vi "FT-IR Kalibrieren Linearisierung.vi"(6 "Kalibrier Optionen:":enum32{"Gasteiler", "ohne Gasteiler", "PNS"}(ring), 9 "Sprachliste":string[][](array[string]), 10 "reference (Eingang)":refnum<vi>, 11 "String (Eingang)":refnum<vi>) -> ()   [LabVIEW 2020, in "Linearisierung v2.lvlib"]
uses:
  Linearisierung v2.lvlib
  Gasteiler/Aktionen FGV Gasteiler Daten.ctl
  Gasteiler/AK-Komm Gasteiler/Aktionen AK Komm.ctl
  Aktion Lin Daten aufarbeiten.ctl
  Gasteiler/Horiba/Aktion Befehl.ctl
  Gasteiler/AK-Komm Gasteiler/Alter Gasteiler/Aktionen AK Komm_ALT.ctl
  Funktionstasten/Funktionstasten-Aktion.ctl
  Funktionstasten/Zustaende.ctl
  Sprachverwaltung/Sprachverwaltung.lvlib
  Gasteiler/Gasteiler.lvlib
  Gasteiler/AK-Komm Gasteiler/AK Komm Gasteiler.lvlib
  Gasteiler/Horiba/Horiba GDC.lvlib
  Gasteiler/AK-Komm Gasteiler/Alter Gasteiler/Alter Gasteiler.lvlib
  Funktionstasten/Funktionstasten.lvlib
  Allgemein/allgemeine Sub-VIs.lvlib
  Gasteiler/HovaCAL_Interface/Kommunikation/Kommunikation.lvlib
  Gasteiler/HovaCAL_Interface/Helper/Helper.lvlib
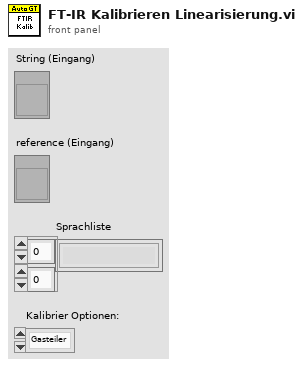
[diagram p1: front panel]
types:
  T1 = typedef "Linearisierung v2.lvlib/Gasteiler.lvlib/Aktionen FGV Gasteiler Daten.ctl" = enum16{"lesen", "Gasteiler Daten", "Seriellen Param.", "MB-Endwert", "laden", "speichern", "Anforderung", "TCP", "Aufzeichnung Start"}
  T2 = typedef "Linearisierung v2.lvlib/Gasteiler.lvlib/AK Komm Gasteiler.lvlib/Aktionen AK Komm.ctl" = enum16{"lesen", "initialisieren", "beenden", "Status", "SMAN", "SREM", "STBY", "ASTF", "ASTZ", "SLST", "AGAT", "EGAK", "AGAK", "AKAK", "ADRU", "SKOP", "SVSA", "SVSZ", "SONO", "SAIR", "SNOX", "ANOX", "SSPL", "SRUC", "SLIN", "ALST", "ETYP", "SVIO", "LCYL", "CCYL", "DCYL", "SCYL", "GCYL", "DRGV", "DRDC"}
  T3 = typedef "Linearisierung v2.lvlib/Aktion Lin Daten aufarbeiten.ctl" = enum16{"lesen", "Protkolldaten", "speichern", "laden", "EPA auswerten", "Tabelle schreiben", "Lin auswerten", "Tab init", "Stufentabelle", "EPA aktiviert", "Nachbehandlung laden", "Tabelle löschen", "Istwerte löschen", "Zeile löschen", "Zeile einfügen", "LIN aktiviert", "LIN/EPA aktiv laden", "EGAK Tab", "LIN übernehmen", "Tab init ohne Stufen"}
  T4 = typedef "Linearisierung v2.lvlib/Gasteiler.lvlib/Horiba GDC.lvlib/Aktion Befehl.ctl" = enum16{"lesen", "initialisieren", "Beenden", "Standby", "GD/CC", "Info", "Flow", "Alarm", "GD parameter", "GD point", "Durchfluss", "Spuelen1", "Spuelen1 On", "Spuelen1Off", "Spuelen2", "Ventil-Abfrage", "Reset"}
  T5 = typedef "Linearisierung v2.lvlib/Gasteiler.lvlib/AK Komm Gasteiler.lvlib/Alter Gasteiler.lvlib/Aktionen AK Komm_ALT.ctl" = enum16{"lesen", "initialisieren", "beenden", "SRES", "STBY", "SREM", "SMAN", "SLIN", "SLCH", "SLST", "SSPL", "AGAT", "ALST", "ASTZ", "ASTF", "AGAK", "EGAK"}
  T6 = typedef "Funktionstasten.lvlib/Funktionstasten-Aktion.ctl" = enum16{"Initialisieren", "Zustand setzen", "Taste gedrückt", "Fehler speichern", "Lesen", "Manuell", "Remote", "Bitparallel", "Samplepoint", "Zeit Prüfen", "reset Umschalten"}
  T7 = typedef "Funktionstasten.lvlib/Zustaende.ctl" = enum16{"Standby", "Pause", "Eco", "Messen", "Kalibrieren", "Spülen Filter", "Spülen Leitung", "Umgebungsluft", "0-Gas", "Cal-Gas", "CG zu PNS", "-------------", "Init 1", "Init 2", "Init 3", "Init 4", "Messen vorbereiten", "Messen durchführen", "Exit"}
  T8 = typedef "Linearisierung v2.lvlib/GasteilerType.ctl" = u16
  T9 = typedef "Linearisierung v2.lvlib/Lin-Polynom Daten.ctl" = cluster{"Messgerät":string, "Kalibrator (Gasteiler)":string, "Bearbeiter/in":string, "Komponente":string, "Zeitstempel":timestamp, "F_max gefordert (%)":sgl, "F_max in %":sgl, "F_max in ppm":sgl, "Vorschlag Ordnung":i32, "Polynom OK":bool, "Polynomkoeff.":dbl[], "Prüfgas Konzentration":dbl, "Pfad EPA":string, "Pfad_LIN":string, "Gasnummer:":u8, "Komponentenauswahl":T10, "Verdünnungsgas":T12, "Zeitdauer Stufe":T13, "Anzahl Stufen":T13, "F_max in % EPA":sgl, "F_max in ppm EPA":sgl, "F_max in % LIN":sgl, "F_max in ppm LIN":sgl, "Punkte umkehren":bool, "EPA Optionsfeld":T14, "Autolin Hovacal":T15, "Spanfactors":sgl[], "Kalibrierauswahl":T16, "Conditions:":T17, "Gasflaschen Nr.:":string, "Bottle Accuracy":dbl, "Konfig Gasflasche":T18, "Gasflasche":T19, "HovaCAL Flow AutoLin":T20, "MFC Output":T21, "Gas Ablaufdatum":timestamp, "Lin Modus":T22, "zusätzliche Zeitdauer Erster Punkt":sgl, "Offsets":sgl[]}
  T10 = typedef "Linearisierung v2.lvlib/KomponentenArray.ctl" = cluster{"Komponente:":T11, "Konzentration":dbl}[]
  T11 = typedef "Auswahlfeld.ctl" = u16
  T12 = typedef "Linearisierung v2.lvlib/Gasteiler.lvlib/Prüfgas in.ctl" = u16
  T13 = typedef "Zahlen-Eingabefeld.ctl" = sgl
  T14 = typedef "Linearisierung v2.lvlib/EPA Optionsfeld.ctl" = enum32{"Istwert", "Rohwert", "Linearisierter Wert"}
  T15 = typedef "Linearisierung v2.lvlib/Gasteiler.lvlib/HovaCal.lvlib/AutoLin Hovacal.ctl" = enum32{"Keine Auswahl", "Optionsauswahl 1", "Optionsauswahl 2"}
  T16 = typedef "Linearisierung v2.lvlib/Kalibrieroption.ctl" = u16
  T17 = typedef "Linearisierung v2.lvlib/Linearity verification 1065-307.lvlib/Condition.ctl" = u16
  T18 = typedef "System Einstellungen V2.lvlib/Konfig Gasflasche.ctl" = bool
  T19 = typedef "System Einstellungen V2.lvlib/Gasflasche Auswahl.ctl" = u16
  T20 = typedef "Linearisierung v2.lvlib/Gasteiler.lvlib/HovaCAL_Interface.lvlib/Controls.lvlib/Flow Einstellung.ctl" = cluster{"HovaCAL Flow Input Cluster":dbl}
  T21 = typedef "Linearisierung v2.lvlib/Gasteiler.lvlib/HovaCAL_Interface.lvlib/Controls.lvlib/Pump state.ctl" = cluster{"Run":bool}
  T22 = typedef "CalGas Aufschaltung.lvlib/Lin Modus.ctl" = u16
  T23 = typedef "Button.ctl" = bool
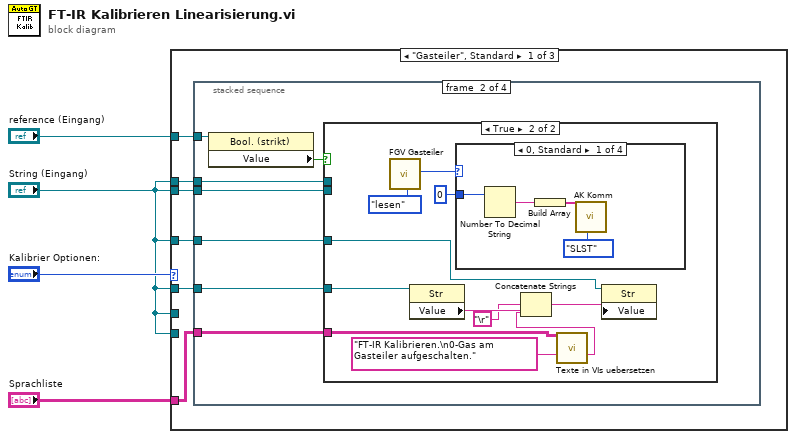
[diagram p0: block diagram]
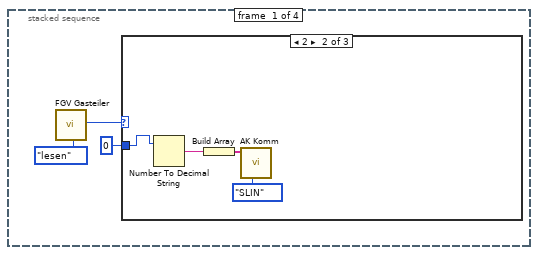
[diagram p2: hidden frame]
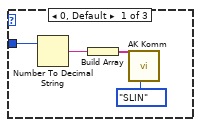
[diagram p3: hidden frame]
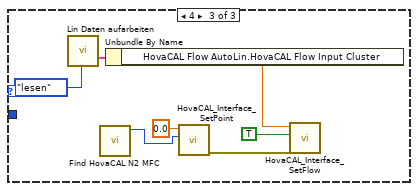
[diagram p4: hidden frame]
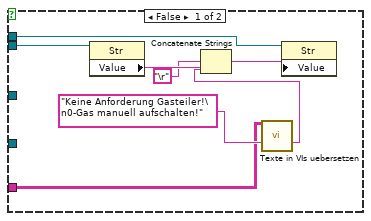
[diagram p5: hidden frame]
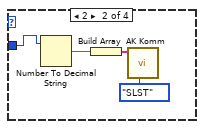
[diagram p6: hidden frame]
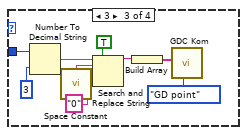
[diagram p7: hidden frame]
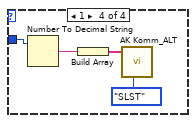
[diagram p8: hidden frame]
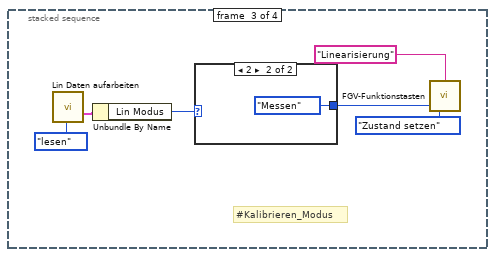
[diagram p9: hidden frame]
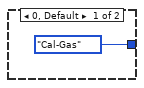
[diagram p10: hidden frame]
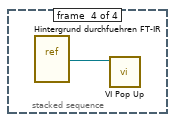
[diagram p11: hidden frame]
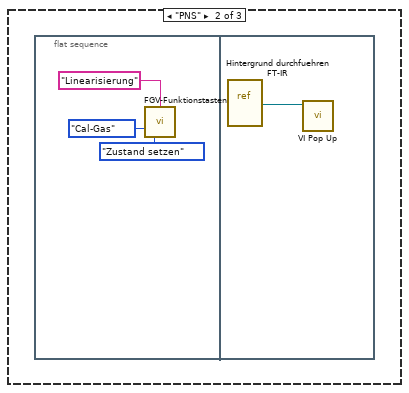
[diagram p12: hidden frame]
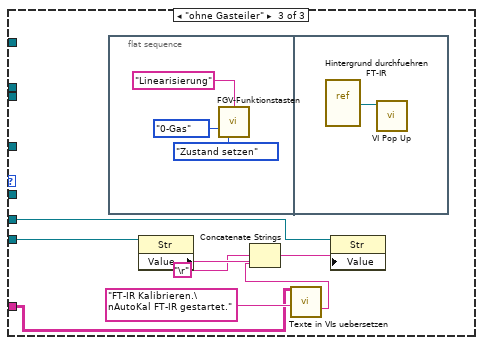
[diagram p13: hidden frame]
diagram:
  n1 = case shown="\"Gasteiler\", Standard" "Kalibrier Optionen:" {
    tunnel: "Sprachliste" -> [w10 _ w91]
    tunnel: "String (Eingang)" -> [w9 _ _]
    tunnel: "String (Eingang)" -> [w8 _ _]
    tunnel: "String (Eingang)" -> [w7 _ _]
    tunnel: "String (Eingang)" -> [w6 _ _]
    tunnel: "reference (Eingang)" -> [w5 _ _]
    tunnel: "String (Eingang)" -> [_ _ w90]
    tunnel: "String (Eingang)" -> [_ _ w89]
    frame "Gasteiler", Default {
      n2 = stacked-sequence {
        tunnel: w10 -> [_ w34 _ _]
        tunnel: w9 -> [_ w33 _ _]
        tunnel: w8 -> [_ w32 _ _]
        tunnel: w7 -> [_ w31 _ _]
        tunnel: w6 -> [_ w30 _ _]
        tunnel: w5 -> [_ w29 _ _]
        frame #0 {
          n3 = call "FGV Gasteiler.vi"("Aktionen"=Aktionen_FGV_Gasteiler_Daten."lesen") -> ("Gasteiler Type"=w13:T8)  [unwired: 11 in, 7 out]
          n4 = case shown="2" w13 {
            tunnel: 0 ("Punkt") -> [w14 w20 _]
            frame 0, Default {
              n5 = Number To Decimal String(number=w14) -> (decimal integer string=w17:string)  [unwired: 1 in]
              n6 = Build Array(w17) -> (w16:string[])
              n7 = call "AK Komm.vi"("Aktionen"=Aktionen_AK_Komm."SLIN", "Daten"=w16) -> ()  [unwired: 3 in, 7 out]
            }
            frame 2 {
              n8 = Number To Decimal String(number=w20) -> (decimal integer string=w21:string)  [unwired: 1 in]
              n9 = Build Array(w21) -> (w19:string[])
              n10 = call "AK Komm.vi"("Aktionen"=Aktionen_AK_Komm."SLIN", "Daten"=w19) -> ()  [unwired: 3 in, 7 out]
            }
            frame 4 {
              n11 = call "Lin Daten aufarbeiten.vi"("Aktionen"=Aktion_Lin_Daten_aufarbeiten."lesen") -> ("Lin-Polynom"=w27:T9)  [unwired: 16 in, 10 out]
              n12 = call "Find HovaCAL N2 MFC.vi"() -> ("N2 MFC Idx"=w22:i32)  [unwired: 11 in]
              n13 = Unbundle By Name(w27) -> ("HovaCAL Flow AutoLin.HovaCAL Flow Input Cluster"=w24:dbl)
              n14 = call "HovaCAL_Interface_SetPoint.vi"("AutoLin MFC Index"=w22, "Konzentration"=0.0) -> ("error out"=w23:errorcluster)  [unwired: 9 in]
              n15 = call "HovaCAL_Interface_SetFlow.vi"("error in (no error)"=w23, "sofort"=TRUE, "total flow setpoint"=w24) -> ()  [unwired: 8 in, 1 out]
            }
          }
        }
        frame #1 {
          n16 = property class="Bool. (strikt)"(reference=w29) -> ("Value"=w35:T23)  [unwired: 1 in, 2 out]
          n17 = case shown="True" w35 {
            tunnel: w34 -> [w38 w46]
            tunnel: w33 -> [w37 _]
            tunnel: w32 -> [w36 _]
            tunnel: w31 -> [_ w45]
            tunnel: w30 -> [_ w44]
            frame False {
              n18 = property class="Str"(reference=w37) -> ("Value"=w43:string)  [unwired: 1 in, 2 out]
              n19 = call "Texte in VIs uebersetzen.vi"("Sprachliste"=w38, "String zum Übersetzen"="Keine Anforderung Gasteiler!\n0-Gas manuell aufschalten!" ("String")) -> ("String zum Übersetzen"=w39:string)  [unwired: 9 in, 4 out]
              n20 = Concatenate Strings(w43, "\r", w39) -> (w42:string)
              n21 = property class="Str"(reference=w36, "Value"=w42) -> ()  [unwired: 1 in, 2 out]
            }
            frame True {
              n22 = call "FGV Gasteiler.vi"("Aktionen"=Aktionen_FGV_Gasteiler_Daten."lesen") -> ("Gasteiler Type"=w54:T8)  [unwired: 11 in, 7 out]
              n23 = property class="Str"(reference=w45) -> ("Value"=w51:string)  [unwired: 1 in, 2 out]
              n24 = case shown="0, Standard" w54 {
                tunnel: 0 ("Punkt") -> [w55 w61 w69 w74]
                frame 0, Default {
                  n25 = Number To Decimal String(number=w55) -> (decimal integer string=w58:string)  [unwired: 1 in]
                  n26 = Build Array(w58) -> (w57:string[])
                  n27 = call "AK Komm.vi"("Aktionen"=Aktionen_AK_Komm."SLST", "Daten"=w57) -> ()  [unwired: 3 in, 7 out]
                }
                frame 2 {
                  n28 = Number To Decimal String(number=w61) -> (decimal integer string=w62:string)  [unwired: 1 in]
                  n29 = Build Array(w62) -> (w60:string[])
                  n30 = call "AK Komm.vi"("Aktionen"=Aktionen_AK_Komm."SLST", "Daten"=w60) -> ()  [unwired: 3 in, 7 out]
                }
                frame 3 {
                  n31 = Number To Decimal String(number=w69, width (-)=i16 3 ("Breite (-)")) -> (decimal integer string=w64:string)
                  n32 = call <vilib>:"Space Constant.vi"() -> ("String"=w68:string)
                  n33 = Search and Replace String(replace all?=TRUE ("Alle ersetzen? (F)"), input string=w64, search string=w68, replace string="0" ("Ersetzungs-String (\"\")")) -> (result string=w65:string)  [unwired: 4 in, 3 out]
                  n34 = Build Array(w65) -> (w70:string[])
                  n35 = call "GDC Kom.vi"("Befehl"=Aktion_Befehl."GD point", "Daten"=w70) -> ()  [unwired: 3 in, 7 out]
                }
                frame 1 {
                  n36 = Number To Decimal String(number=w74) -> (decimal integer string=w75:string)  [unwired: 1 in]
                  n37 = Build Array(w75) -> (w73:string[])
                  n38 = call "AK Komm_ALT.vi"("Aktionen_ALT"=Aktionen_AK_Komm_ALT."SLST", "Daten"=w73) -> ()  [unwired: 5 in, 5 out]
                }
              }
              n39 = call "Texte in VIs uebersetzen.vi"("Sprachliste"=w46, "String zum Übersetzen"="FT-IR Kalibrieren.\n0-Gas am Gasteiler aufgeschalten." ("String")) -> ("String zum Übersetzen"=w47:string)  [unwired: 9 in, 4 out]
              n40 = Concatenate Strings(w51, "\r", w47) -> (w50:string)
              n41 = property class="Str"(reference=w44, "Value"=w50) -> ()  [unwired: 1 in, 2 out]
            }
          }
        }
        frame #2 {
          # "#Kalibrieren_Modus"
          n42 = call "Lin Daten aufarbeiten.vi"("Aktionen"=Aktion_Lin_Daten_aufarbeiten."lesen") -> ("Lin-Polynom"=w78:T9)  [unwired: 16 in, 10 out]
          n43 = Unbundle By Name(w78) -> ("Lin Modus"=w77:T22)
          n44 = case shown="2" w77 {
            tunnel: [Zustaende."Cal-Gas" ("Zustand") Zustaende."Messen" ("Zustand")] -> w76
            frame 0, Default {
            }
            frame 2 {
            }
          }
          n45 = call "FGV-Funktionstasten.vi"("Herkunft"="Linearisierung", "Zustand"=w76, "Aktion"=Funktionstasten-Aktion."Zustand setzen") -> ()  [unwired: 5 in, 8 out]
        }
        frame #3 {
          n46 = vi-ref "Hintergrund durchfuehren FT-IR.vi"() -> (w84:refnum<vi>)
          n47 = call "VI Pop Up.vi"("VI Referenz"=w84) -> ()  [unwired: 10 in, 1 out]
        }
      }
    }
    frame "PNS" {
      n48 = flat-sequence {
        frame #0 {
          n49 = call "FGV-Funktionstasten.vi"("Herkunft"="Linearisierung", "Zustand"=Zustaende."Cal-Gas", "Aktion"=Funktionstasten-Aktion."Zustand setzen") -> ()  [unwired: 5 in, 8 out]
        }
        frame #1 {
          n50 = vi-ref "Hintergrund durchfuehren FT-IR.vi"() -> (w88:refnum<vi>)
          n51 = call "VI Pop Up.vi"("VI Referenz"=w88) -> ()  [unwired: 10 in, 1 out]
        }
      }
    }
    frame "ohne Gasteiler" {
      n52 = flat-sequence {
        frame #0 {
          n53 = call "FGV-Funktionstasten.vi"("Herkunft"="Linearisierung", "Zustand"=Zustaende."0-Gas", "Aktion"=Funktionstasten-Aktion."Zustand setzen") -> ()  [unwired: 5 in, 8 out]
        }
        frame #1 {
          n54 = vi-ref "Hintergrund durchfuehren FT-IR.vi"() -> (w100:refnum<vi>)
          n55 = call "VI Pop Up.vi"("VI Referenz"=w100) -> ()  [unwired: 10 in, 1 out]
        }
      }
      n56 = property class="Str"(reference=w90) -> ("Value"=w96:string)  [unwired: 1 in, 2 out]
      n57 = call "Texte in VIs uebersetzen.vi"("Sprachliste"=w91, "String zum Übersetzen"="FT-IR Kalibrieren.\nAutoKal FT-IR gestartet." ("String")) -> ("String zum Übersetzen"=w92:string)  [unwired: 9 in, 4 out]
      n58 = Concatenate Strings(w96, "\r", w92) -> (w95:string)
      n59 = property class="Str"(reference=w89, "Value"=w95) -> ()  [unwired: 1 in, 2 out]
    }
  }
